vi "固件升级（包含参数恢复）.vi"(10 "路径对话框":bool, 11 "selected path":path) -> (3 "结果字符串":string)   [LabVIEW 2022 SP3, in "斯坦道通用流路CODmn.lvlib"]
uses:
  <vilib>/NI/Progress Bar/Controls/Progress Bar Properties.ctl
  <vilib>/Utility/error.llb/DialogType.ctl
  <vilib>/NI/Progress Bar/Progress Bar.lvlib
panel:
  out "布尔":bool
  out "仪器公式":T1(array[cluster])
  out "量程参数":T2(array[cluster])
  out "试剂容量参数":T3
  out "外设参数":cluster{"仪器版本":T4, "error out":errorcluster}
  out "固件升级步骤":T5
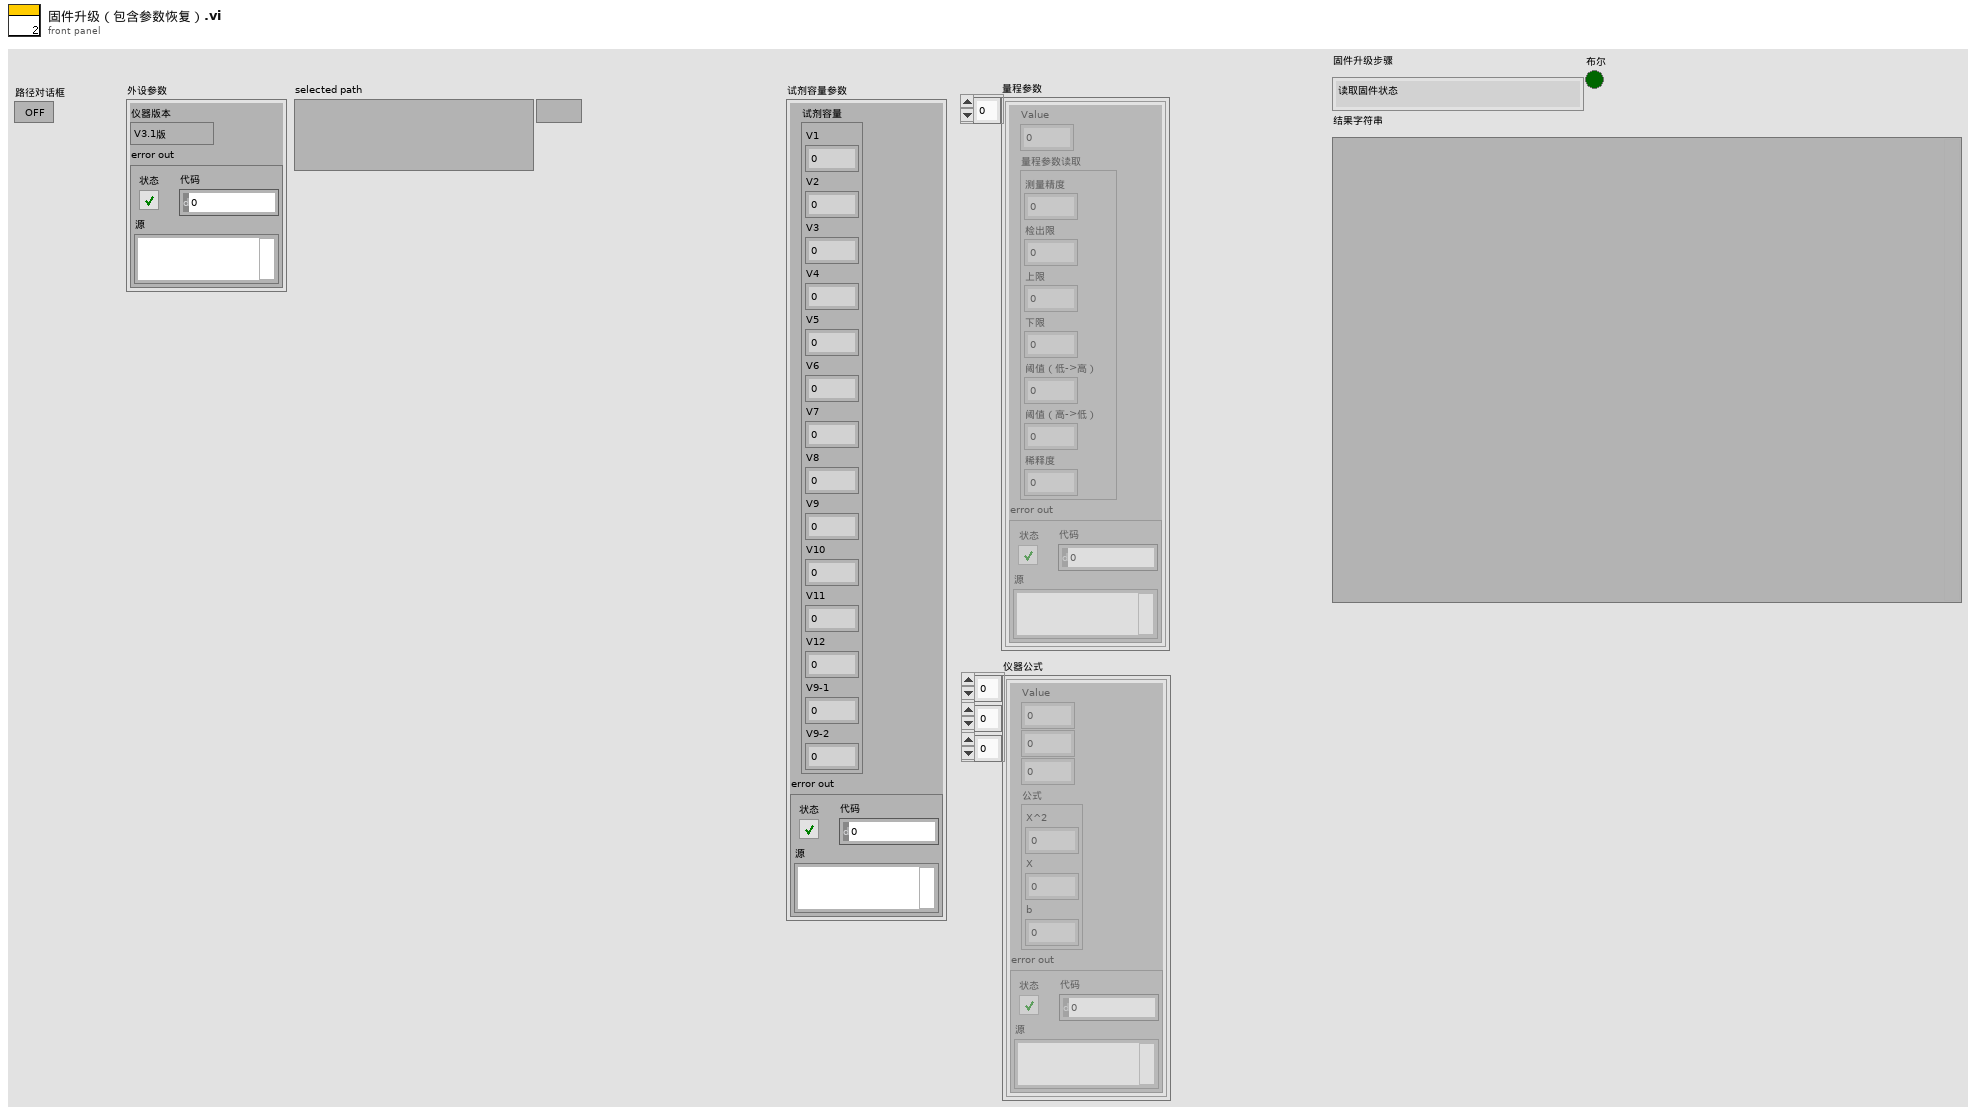
[diagram p1: front panel]
types:
  T1 = cluster{"Value":u16, i32, i32, "公式":cluster{"X^2":dbl, "X":dbl, "b":dbl}, "error out":errorcluster}[][][]
  T2 = cluster{"Value":u16, "量程参数读取":cluster{"测量精度":u16, "检出限":dbl, "上限":dbl, "下限":dbl, "阈值（低->高）":dbl, "阈值（高->低）":dbl, "稀释度":dbl}, "error out":errorcluster}[]
  T3 = cluster{"试剂容量":cluster{"V1":sgl, "V2":sgl, "V3":sgl, "V4":sgl, "V5":sgl, "V6":sgl, "V7":sgl, "V8":sgl, "V9":sgl, "V10":sgl, "V11":sgl, "V12":sgl, "V9-1":sgl, "V9-2":sgl}, "error out":errorcluster}
  T4 = typedef "SingleStepTestV3.lvlib/SingleStepTestV3.lvclass/仪器版本.ctl" = enum16{"V3.1版", "V4版", "V3版", "V4.2版"}
  T5 = typedef "斯坦道通用流路CODmn.lvlib/固件升级步骤.ctl" = enum16{"读取固件状态", "备份参数", "写入仪器固件", "恢复参数", "询问是否写入流程", "写入测试流程", "结束"}
  T6 = typedef "Progress Bar.lvlib/Progress Bar Properties.ctl" = cluster{"Background Color":u32, "Installer Title":string, "Title Color":u32, "Action Text":string, "Text Color":u32, "Slider Value":u8, "Bar Color":u32, "Timeout":i32}
  T7 = typedef "DialogType.ctl" = u16
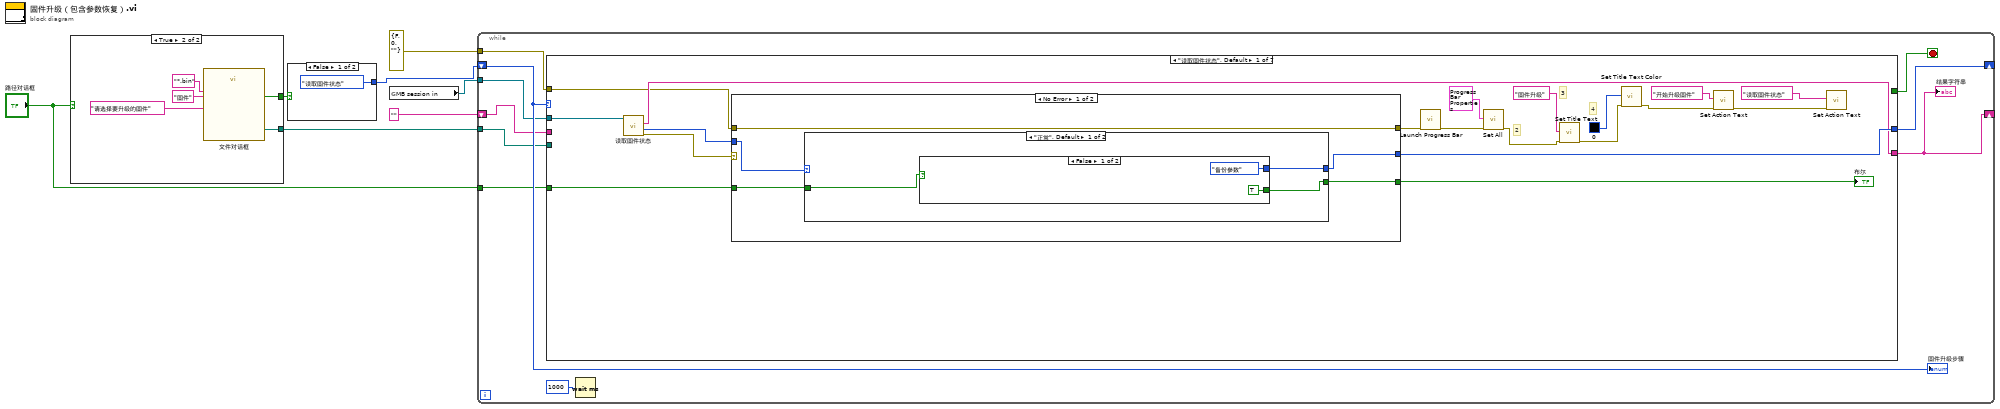
[diagram p0: block diagram]
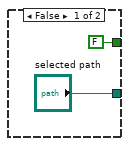
[diagram p2: hidden frame]
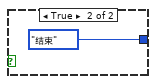
[diagram p3: hidden frame]
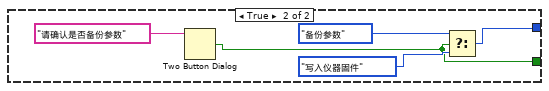
[diagram p4: hidden frame]
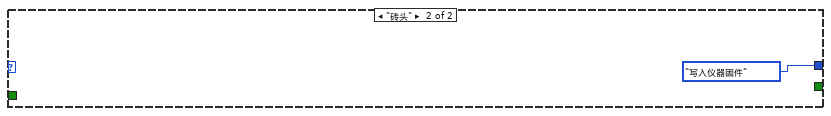
[diagram p5: hidden frame]
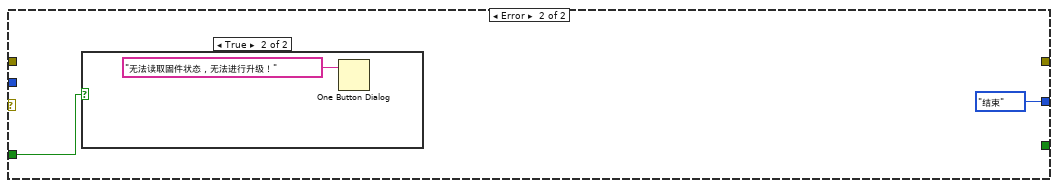
[diagram p6: hidden frame]
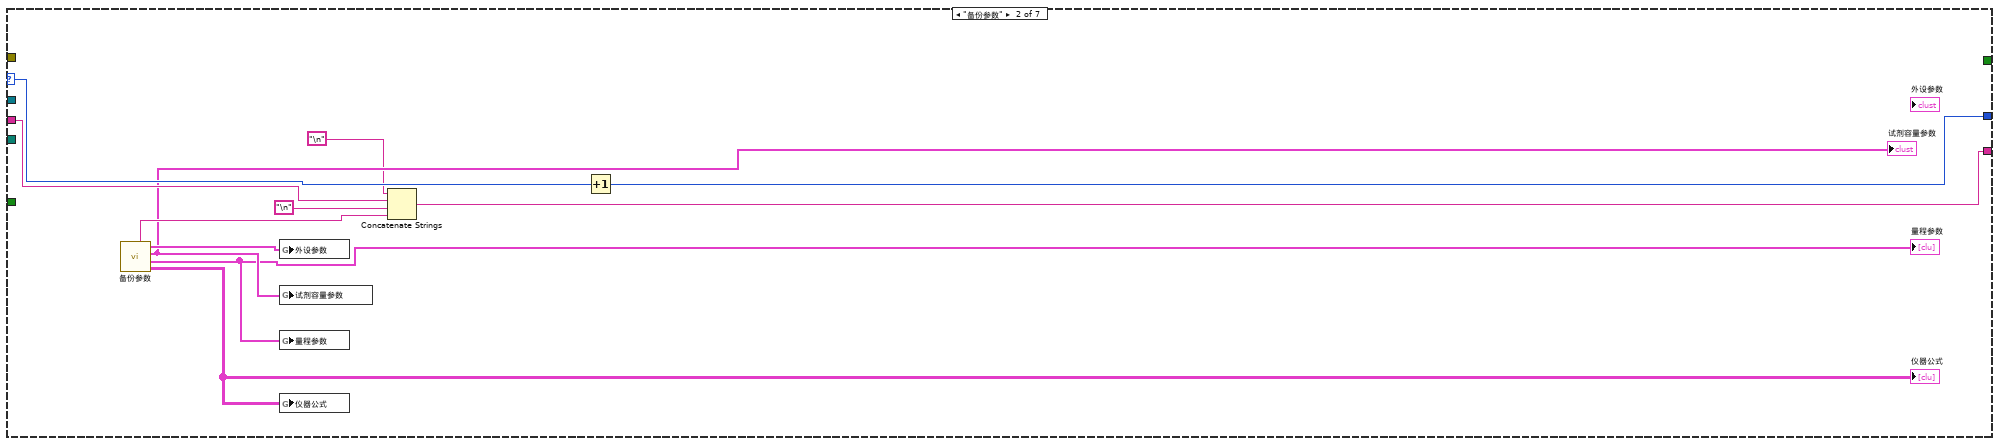
[diagram p8: hidden frame]
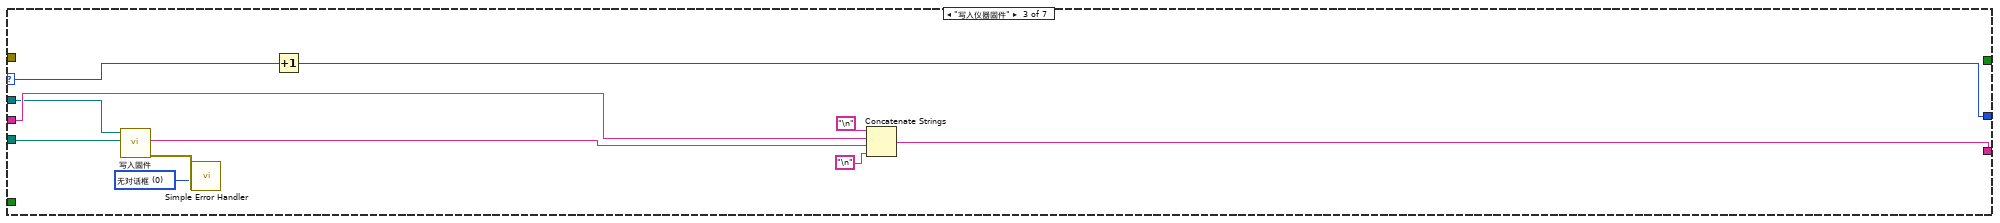
[diagram p9: hidden frame]
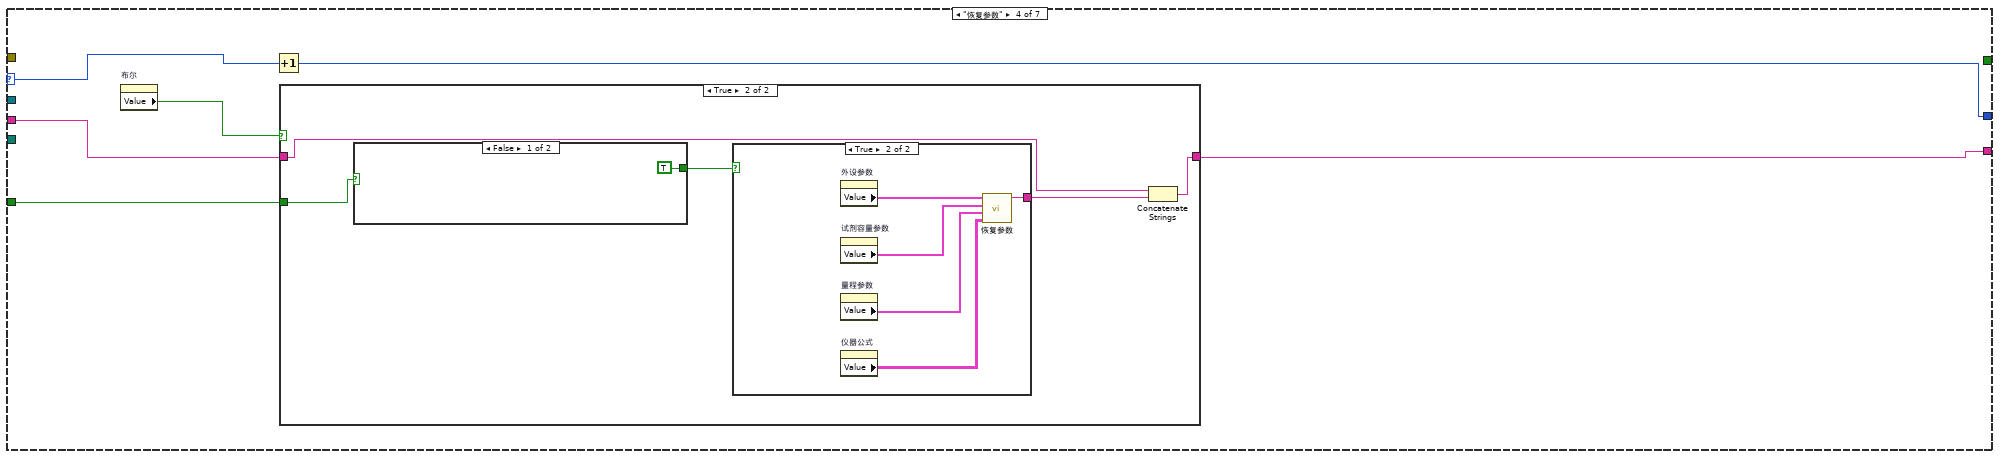
[diagram p10: hidden frame]
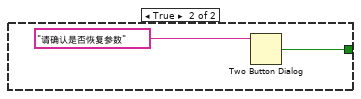
[diagram p12: hidden frame]
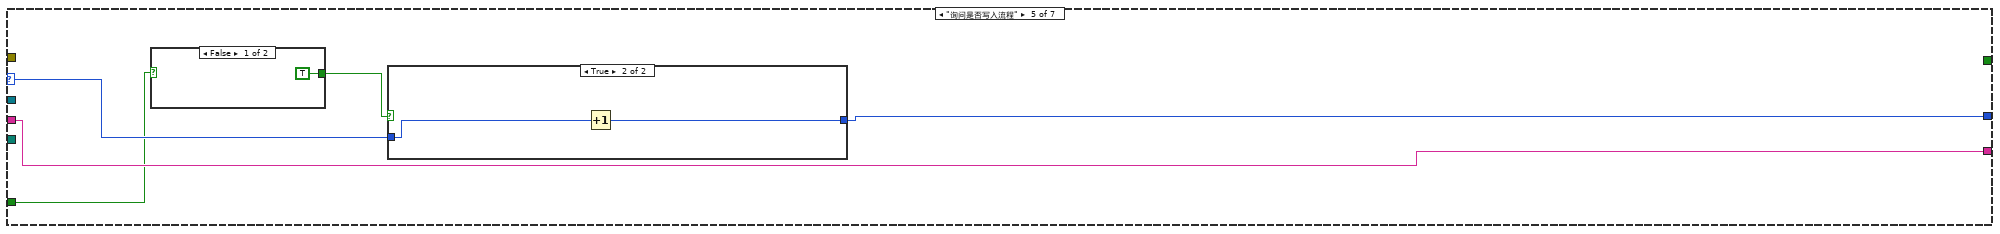
[diagram p14: hidden frame]
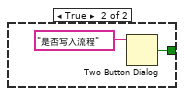
[diagram p15: hidden frame]
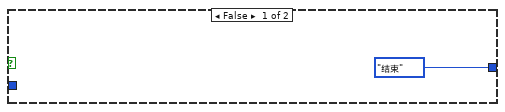
[diagram p16: hidden frame]
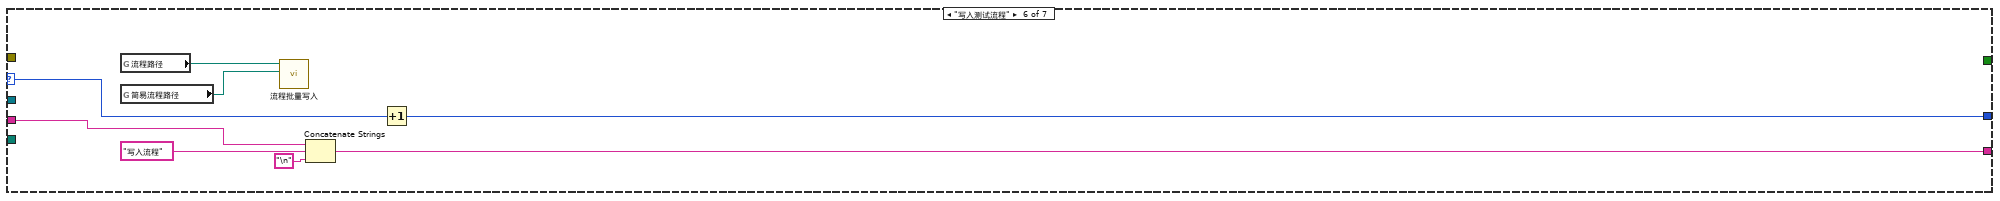
[diagram p17: hidden frame]
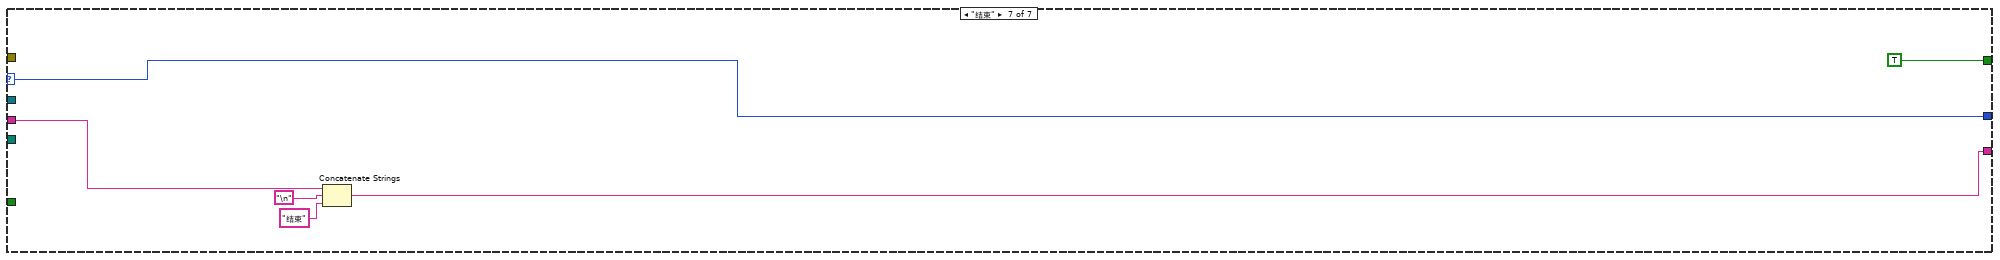
[diagram p18: hidden frame]
diagram:
  n1 = case shown="True" "路径对话框" {
    tunnel: ["selected path" w11] -> w5
    tunnel: [FALSE ("cancelled") w10] -> w3
    frame False {
    }
    frame True {
      n2 = call "文件对话框"("prompt"="请选择要升级的固件", "pattern (all files)"="*.bin", "pattern label"="固件") -> ("selected path"=w11:path, "cancelled"=w10:bool)  [unwired: 9 in, 2 out]
    }
  }
  n3 = case shown="False" w3 {
    tunnel: [固件升级步骤."读取固件状态" ("固件升级步骤") 固件升级步骤."结束" ("固件升级步骤")] -> w4
    frame False {
    }
    frame True {
    }
  }
  n4 = global read "VAR总磷总氮全局变量.vi" "MB session in"() -> (w7:refnum<class "MB_Master.lvclass">)
  n5 = while {
    tunnel: w7 -> [w25]
    shift-right: [w24] -> _
    shift-left: w4 -> [w26]
    shift-right: [w20] -> _
    shift-left: "" ("结果字符串") -> [w21]
    tunnel: w5 -> [w19]
    tunnel: errorcluster {"status"=FALSE, "code"=0, "source"=""} ("error out") -> [w18]
    tunnel: "路径对话框" -> [w17]
    stop <- w23 stop-if-true
    n6 = case shown="\"读取固件状态\", Default" w26 {
      selector: w26 -> [_ w75 w86 w89 w110 w123 w130]
      tunnel: w25 -> [w45 _ w82 _ _ _ _]
      tunnel: [w42 w74 w85 w88 w109 w122 w130] -> w24
      tunnel: [_ _ _ _ _ _ TRUE] -> w23
      tunnel: [w41 w73 w83 w91 w108 w120 w126] -> w20
      tunnel: w21 -> [_ w72 w84 w92 w108 w121 w127]
      tunnel: w18 -> [w29 _ _ _ _ _ _]
      tunnel: w19 -> [_ _ w81 _ _ _ _]
      tunnel: w17 -> [w27 _ _ w87 w107 _ _]
      frame "读取固件状态", Default {
        # "4"
        # "3"
        # "2"
        n7 = call "读取固件状态.vi"("MB session in"=w45) -> ("error out"=w43:errorcluster, "固件状态"=w44:enum16{"正常", "砖头"}, "结果字符串"=w41:string)  [unwired: 7 in, 1 out]
        n8 = case shown="No Error" w43 {
          tunnel: w44 -> [w50 _]
          tunnel: [w49 固件升级步骤."结束" ("固件升级步骤")] -> w42
          tunnel: [w48 _] -> w39
          tunnel: w29 -> [w47 _]
          tunnel: [w47 _] -> w28
          tunnel: w27 -> [w46 w62]
          frame No Error {
            n9 = case shown="\"正常\", Default" w50 {
              tunnel: [w52 固件升级步骤."写入仪器固件" ("固件升级步骤")] -> w49
              tunnel: [w53 _] -> w48
              tunnel: w46 -> [w51 _]
              frame "正常", Default {
                n10 = case shown="False" w51 {
                  tunnel: [TRUE ("T button?") w57] -> w53
                  tunnel: [固件升级步骤."备份参数" ("固件升级步骤") w56] -> w52
                  frame False {
                  }
                  frame True {
                    n11 = Two Button Dialog(message="请确认是否备份参数" ("消息")) -> (T button?=w57:bool)  [unwired: 2 in]
                    n12 = Select(t=固件升级步骤."备份参数" ("固件升级步骤"), s=w57, f=固件升级步骤."写入仪器固件" ("固件升级步骤")) -> (s? t:f=w56:T5)
                  }
                }
              }
              frame "砖头" {
              }
            }
          }
          frame Error {
            n13 = case shown="True" w62 {
              frame False {
              }
              frame True {
                n14 = One Button Dialog(message="无法读取固件状态，无法进行升级！" ("消息")) -> ()  [unwired: 1 in, 1 out]
              }
            }
          }
        }
        "布尔" <- w39
        n15 = call <vilib>:"Launch Progress Bar.vi"("error in (no error)"=w28) -> ("error out"=w36:errorcluster)  [unwired: 9 in, 1 out]
        n16 = call <vilib>:"Set All.vi"("error in (no error)"=w36, "Progress Bar Properties (Default)"=T6 {"Background Color"=3381759, "Installer Title"="Progress", "Title Color"=0, "Action Text"="", "Text Color"=0, "Slider Value"=0, "Bar Color"=6618880, "Timeout"=30000} ("Progress Bar Properties")) -> ("error out"=w33:errorcluster)  [unwired: 9 in]
        n17 = call <vilib>:"Set Title Text.vi"("error in (no error)"=w33, "Installer Title"="固件升级") -> ("error out"=w31:errorcluster)  [unwired: 9 in]
        n18 = call <vilib>:"Set Title Text Color.vi"("error in (no error)"=w31, "Color Box"=u32 0) -> ("error out"=w34:errorcluster)  [unwired: 9 in]
        n19 = call <vilib>:"Set Action Text.vi"("error in (no error)"=w34, "Action Text"="开始升级固件") -> ("error out"=w38:errorcluster)  [unwired: 9 in]
        n20 = call <vilib>:"Set Action Text.vi"("error in (no error)"=w38, "Action Text"="读取固件状态") -> ()  [unwired: 9 in, 1 out]
      }
      frame "备份参数" {
        n21 = call "备份参数.vi"() -> ("仪器公式"=w66:T1, "量程参数"=w67:T2, "试剂容量参数"=w68:T3, "外设参数"=w69:cluster{"仪器版本":T4, "error out":errorcluster}, "备份结果"=w70:string)  [unwired: 7 in]
        "试剂容量参数" <- w68
        "量程参数" <- w67
        "仪器公式" <- w66
        n22 = global write "VAR总磷总氮全局变量.vi" "外设参数"(w69) -> ()
        n23 = global write "VAR总磷总氮全局变量.vi" "试剂容量参数"(w68) -> ()
        n24 = global write "VAR总磷总氮全局变量.vi" "量程参数"(w67) -> ()
        n25 = global write "VAR总磷总氮全局变量.vi" "仪器公式"(w66) -> ()
        n26 = Concatenate Strings("\n", w72, "\n", w70) -> (w73:string)
        n27 = Increment(x=w75) -> (x+1=w74:T5)
      }
      frame "写入仪器固件" {
        w77 = T7 0 items=["无对话框", "确定信息", "继续或停止信息", "确定信息＋警告", "继续/停止+警告"] ("type of dialog (OK msg:1)")
        n28 = call "写入固件.vi"("selected path"=w81, "MB session in"=w82) -> ("error out"=w78:errorcluster, "结果字符串"=w79:string)  [unwired: 7 in, 1 out]
        n29 = call <vilib>:"Simple Error Handler.vi"("type of dialog (OK msg:1)"=w77, "error in (no error)"=w78) -> ()  [unwired: 3 in, 5 out]
        n30 = Increment(x=w86) -> (x+1=w85:T5)
        n31 = Concatenate Strings("\n", w84, w79, "\n") -> (w83:string)
      }
      frame "恢复参数" {
        n32 = property on="布尔" class="Bool (strict)"() -> ("Value"=w90:bool)  [unwired: 2 in, 2 out]
        n33 = Increment(x=w89) -> (x+1=w88:T5)
        n34 = case shown="True" w90 {
          tunnel: w92 -> [w93 w97]
          tunnel: [w93 w96] -> w91
          tunnel: w87 -> [_ w94]
          frame False {
          }
          frame True {
            n35 = case shown="False" w94 {
              tunnel: [TRUE ("T button?") w100] -> w95
              frame False {
              }
              frame True {
                n36 = Two Button Dialog(message="请确认是否恢复参数" ("消息")) -> (T button?=w100:bool)  [unwired: 2 in]
              }
            }
            n37 = case shown="True" w95 {
              tunnel: [_ w102] -> w98
              frame False {
              }
              frame True {
                n38 = property on="外设参数" class="Clust (strict)"() -> ("Value"=w106:cluster{"仪器版本":T4, "error out":errorcluster})  [unwired: 2 in, 2 out]
                n39 = property on="试剂容量参数" class="Clust (strict)"() -> ("Value"=w105:T3)  [unwired: 2 in, 2 out]
                n40 = property on="量程参数" class="Arr (strict)"() -> ("Value"=w104:T2)  [unwired: 2 in, 2 out]
                n41 = property on="仪器公式" class="Arr (strict)"() -> ("Value"=w103:T1)  [unwired: 2 in, 2 out]
                n42 = call "恢复参数.vi"("仪器公式"=w103, "量程参数"=w104, "试剂容量参数"=w105, "外设参数"=w106) -> ("恢复结果"=w102:string)  [unwired: 7 in]
              }
            }
            n43 = Concatenate Strings(w97, w98) -> (w96:string)
          }
        }
      }
      frame "询问是否写入流程" {
        n44 = case shown="False" w107 {
          tunnel: [TRUE ("T button?") w113] -> w111
          frame False {
          }
          frame True {
            n45 = Two Button Dialog(message="是否写入流程" ("消息")) -> (T button?=w113:bool)  [unwired: 2 in]
          }
        }
        n46 = case shown="True" w111 {
          tunnel: w110 -> [_ w117]
          tunnel: [固件升级步骤."结束" w116] -> w109
          frame False {
          }
          frame True {
            n47 = Increment(x=w117) -> (x+1=w116:T5)
          }
        }
      }
      frame "写入测试流程" {
        n48 = global read "总磷总氮断电保存全局变量.vi" "流程路径"() -> (w125:path)
        n49 = global read "总磷总氮断电保存全局变量.vi" "简易流程路径"() -> (w124:path)
        n50 = call "流程批量写入.vi"("简易流程路径"=w124, "添加的路径"=w125) -> ()  [unwired: 10 in]
        n51 = Concatenate Strings(w121, "写入流程" ("字符串"), "\n") -> (w120:string)
        n52 = Increment(x=w123) -> (x+1=w122:T5)
      }
      frame "结束" {
        n53 = Concatenate Strings(w127, "\n", "结束" ("字符串")) -> (w126:string)
      }
    }
    "结果字符串" <- w20
    n54 = Wait (ms)(milliseconds to wait=u32 1000 ("等待时间（毫秒）")) -> ()  [unwired: 1 out]
    "固件升级步骤" <- w26
  }
